vi "Delta Analysis.vi"() -> ()   [LabVIEW 2013]
uses:
  Common/Delta Analyzor/Workspace Scope.ctl
  <vilib>/Math Plots/3D Math Plots/3D Scatter/3D Scatter XCtrl/3D Scatter.xctl
  Common/Delta Analyzor/Delta Analyzor.lvclass
  <vilib>/Analysis/_algsub.llb/Real Vector Norm.vi
  <vilib>/picture/3D Picture Control/Object/Create Object (name).vi
  <vilib>/Math Plots/3D Math Plots/3D Scatter/3D Scatter Datatype/Public/Plot Helper (Vector).vi
  Common/Delta Robot Kinematics/Delta Robot Kinematics.lvclass
  <vilib>/Math Plots/3D Math Plots/3D Scatter/3D Scatter Datatype/3D Scatter Datatype.lvclass
  <vilib>/Analysis/NI_AALPro.lvlib
  <vilib>/picture/3D Picture Control/NI_3D Picture Control.lvlib
panel:
  out "number test points":i32
  out "XY Graph":cluster{dbl[], dbl[]}(graph)
  out "3D Scatter 2":refnum<class "3D Plot Datatype.lvclass">[](xcontrol)
  out "x*y":dbl[][](array[numeric])
  in  "stop":bool
  out "3D Picture":refnum<vi>(3d-picture)
  out "Waveform Chart":dbl[](graph)
  out "velocity time":u32
  out "workspace time (ms)":u32
  out "3D Scatter":refnum<class "3D Plot Datatype.lvclass">[](xcontrol)
  in  "Workspace Scope":T1={"X range"={"min"=-1.0, "max"=1.0}, "Y range"={"min"=-1.0, "max"=1.0}, "Z range"={"min"=-1.2, "max"=-0.2}}
  in  "XYZ Resolution":dbl[](array[numeric])=[0.05, 0.05, 0.05]
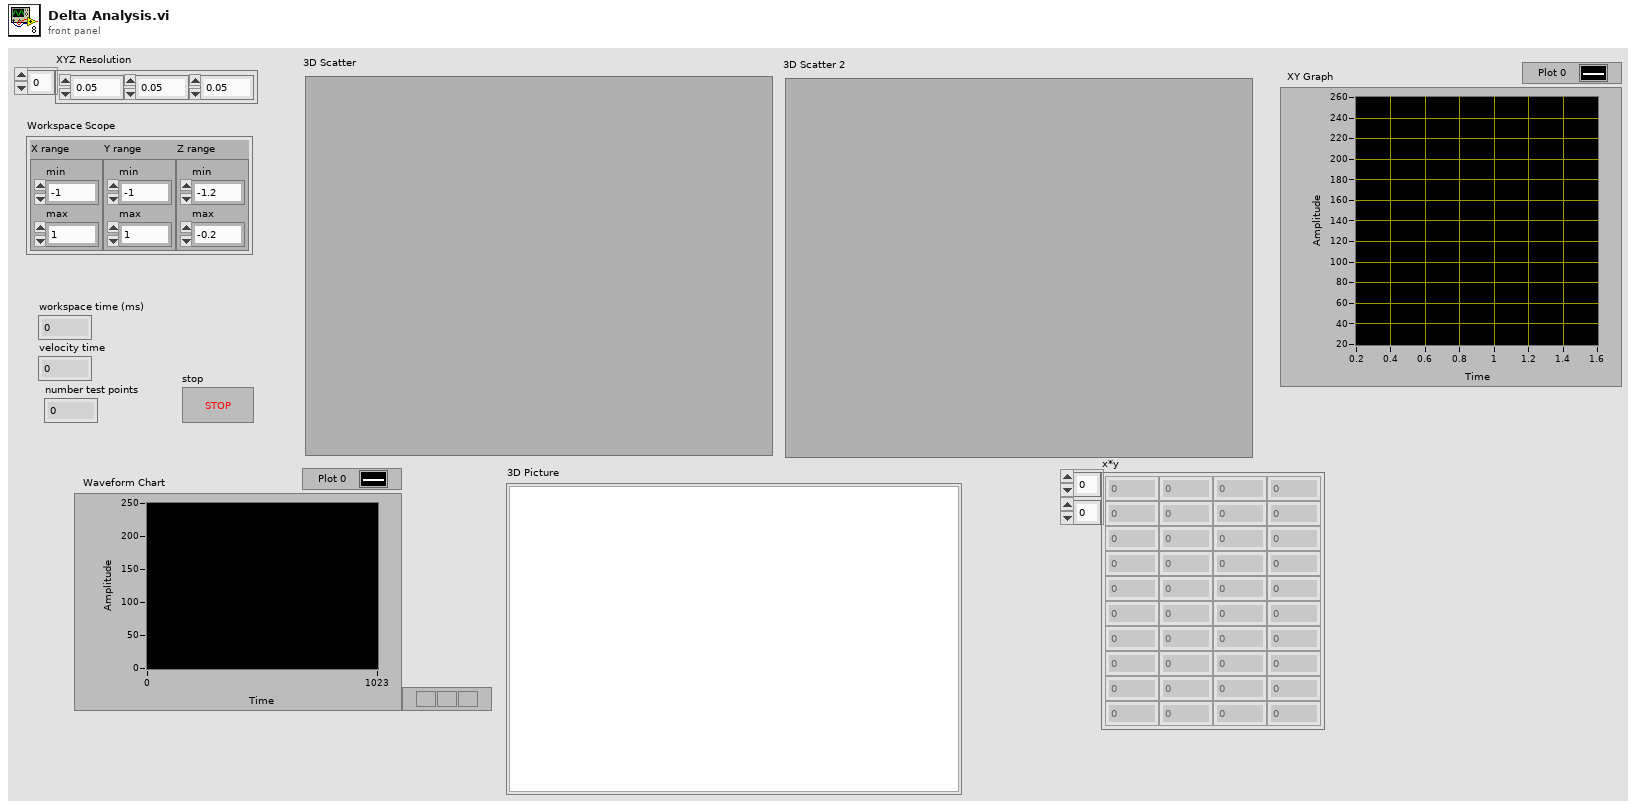
[diagram p1: front panel]
types:
  T1 = typedef "Delta Analyzor.lvclass/Workspace Scope.ctl" = cluster{"X range":cluster{"min":dbl, "max":dbl}, "Y range":cluster{"min":dbl, "max":dbl}, "Z range":cluster{"min":dbl, "max":dbl}}
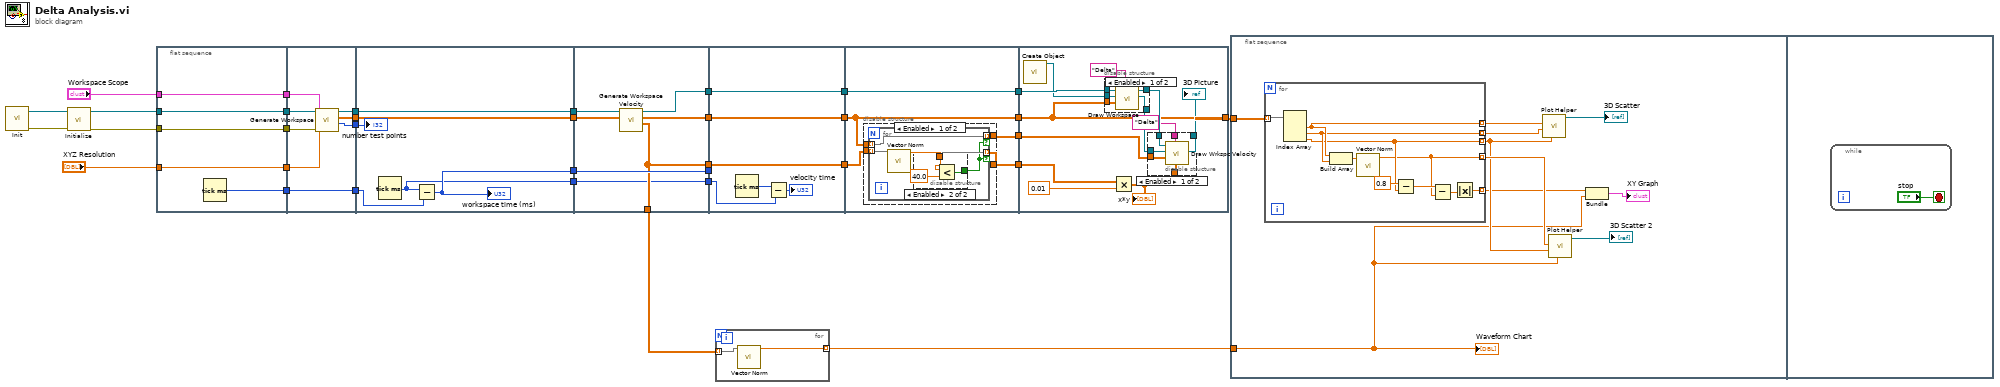
[diagram p0: block diagram]
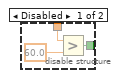
[diagram p2: hidden frame]
diagram:
  n1 = call "Init.vi"() -> ("error out"=w33:errorcluster, "Delta Robot Kin"=w34:refnum<class "Delta Robot Kinematics.lvclass">)  [unwired: 10 in]
  n2 = call "Initialize.vi"("error in (no error)"=w33, "Delta Robot Kinematics"=w34) -> ("error out"=w31:errorcluster, "Delta Analyzor out"=w32:refnum<class "Delta Analyzor.lvclass">)  [unwired: 8 in]
  n3 = flat-sequence {
    tunnel: "Workspace Scope" -> [w36]
    tunnel: "XYZ Resolution" -> [w37]
    tunnel: w31 -> [w38]
    tunnel: w32 -> [w39]
    tunnel: [w39] -> w28
    tunnel: [w38] -> w27
    tunnel: [w37] -> w26
    tunnel: [w36] -> w25
    tunnel: [w35] -> w23
    tunnel: w28 -> [w47]
    tunnel: w27 -> [w46]
    tunnel: w26 -> [w45]
    tunnel: w25 -> [w44]
    tunnel: [w43] -> w24
    tunnel: w23 -> [w42]
    tunnel: [w42] -> w22
    tunnel: [w41] -> w19
    tunnel: [w40] -> w8
    tunnel: w24 -> [w53]
    tunnel: w22 -> [w52]
    tunnel: [w53] -> w21
    tunnel: w19 -> [w51]
    tunnel: [w51] -> w18
    tunnel: [w50] -> w17
    tunnel: [w49] -> w9
    tunnel: w8 -> [w48]
    tunnel: w21 -> [w59]
    tunnel: [w58] -> w20
    tunnel: w18 -> [w60]
    tunnel: w17 -> [w57]
    tunnel: [w57] -> w16
    tunnel: [w55] -> w15
    tunnel: [w56] -> w12
    tunnel: [w55] -> w11
    tunnel: [w54] -> w10
    tunnel: w9 -> [w54]
    tunnel: w20 -> [w66]
    tunnel: w16 -> [_]
    tunnel: [w66] -> w7
    tunnel: w12 -> [w63]
    tunnel: [w63] -> w5
    tunnel: w11 -> [w62]
    tunnel: [w62] -> w3
    tunnel: w10 -> [w61]
    tunnel: w7 -> [w69]
    tunnel: [w69] -> w6
    tunnel: w5 -> [w71]
    tunnel: [w71] -> w4
    tunnel: w3 -> [w70]
    tunnel: [w67] -> w2
    tunnel: [w68] -> w1
    tunnel: [w94] -> w13
    tunnel: w6 -> [w94]
    tunnel: w4 -> [w99]
    tunnel: w2 -> [w91]
    tunnel: w1 -> [w88]
    frame #0 {
      n4 = Tick Count (ms)() -> (millisecond timer value=w35:u32)
    }
    frame #1 {
      n5 = call-dynamic "Generate Workspace.vi"("error in (no error)"=w46, "XYZ Resolution"=w45, "Workspace Scope"=w44, "Delta Analyzor in"=w47) -> ("number test points"=w40:i32, "workspace"=w43:dbl[][], "Delta Analyzor out"=w41:refnum<class "Delta Analyzor.lvclass">)  [unwired: 4 in, 1 out]
    }
    frame #2 {
      n6 = Tick Count (ms)() -> (millisecond timer value=w49:u32)
      n7 = Subtract(x=w49, y=w52) -> (x-y=w50:u32)
      "workspace time (ms)" <- w50
      "number test points" <- w48
    }
    frame #3 {
      n8 = call-dynamic "Generate Workspace Velocity.vi"("workspace in"=w59, "Delta Analyzor in"=w60) -> ("velocities"=w55:dbl[][], "workspace out"=w58:dbl[][], "Delta Analyzor out"=w56:refnum<class "Delta Analyzor.lvclass">)  [unwired: 6 in, 1 out]
    }
    frame #4 {
      n9 = Tick Count (ms)() -> (millisecond timer value=w65:u32)
      n10 = Subtract(x=w65, y=w61) -> (x-y=→"velocity time":u32)
    }
    frame #5 {
      n11 = disable-structure shown="Enabled" {
        disable-tunnel: w70 -> [w75 w86]
        disable-tunnel: w69 -> [w74 w87]
        disable-tunnel: [w73 w87] -> w68
        disable-tunnel: [w72 w86] -> w67
        frame Enabled {
          n12 = for {
            tunnel: w75 -> [w78] mode=indexing
            tunnel: w74 -> [w77] mode=indexing
            tunnel: [w78] -> w72 mode=indexing if=w76
            tunnel: [w77] -> w73 mode=indexing if=w76
            n13 = call-poly <vilib>:"Vector Norm.vi"("Input Vector"=w78) -> ("norm"=w79:dbl)  [unwired: 9 in, 1 out]
            n14 = disable-structure shown="Enabled" {
              disable-tunnel: w79 -> [w81 w85]
              disable-tunnel: [w80 w84] -> w76
              frame Disabled {
                n15 = Greater?(x=w81, y=60.0) -> (0:w80:bool)
              }
              frame Enabled {
                n16 = Less?(x=w85, y=40.0) -> (x < y?=w84:bool)
              }
            }
          }
        }
        frame Disabled {
        }
      }
    }
    frame #6 {
      n17 = call-poly <vilib>:"Create Object.vi"() -> ("Scene:New Object"=w98:refnum<vi>)  [unwired: 10 in, 1 out]
      n18 = disable-structure shown="Enabled" {
        disable-tunnel: w99 -> [w112 w113]
        disable-tunnel: w98 -> [w111 w114]
        disable-tunnel: "Delta" ("name") -> [w110 _]
        disable-tunnel: [w109 w113] -> w96
        disable-tunnel: [w108 w114] -> w95
        disable-tunnel: w94 -> [w107 _]
        frame Enabled {
          n19 = call-dynamic "Draw Workspace.vi"("name"=w110, "workspace in"=w107, "parent sence"=w111, "Delta Analyzor in"=w112) -> ("parent sence out"=w108:refnum<vi>, "Delta Analyzor out"=w109:refnum<class "Delta Analyzor.lvclass">)  [unwired: 4 in, 2 out]
        }
        frame Disabled {
        }
      }
      n20 = Multiply(x=w91, y=0.01) -> (x*y=w90:dbl[][])
      "x*y" <- w90
      n21 = disable-structure shown="Enabled" {
        disable-tunnel: w96 -> [w105 _]
        disable-tunnel: w95 -> [w104 w106]
        disable-tunnel: "Delta" ("name") -> [w103 _]
        disable-tunnel: [w102 w106] -> w92
        disable-tunnel: w90 -> [w101 _]
        disable-tunnel: w88 -> [w100 _]
        frame Enabled {
          n22 = call-dynamic "Draw Wrkspc Velocity.vi"("velocities"=w101, "name"=w103, "workspace in"=w100, "parent sence"=w104, "Delta Analyzor in"=w105) -> ("parent sence out"=w102:refnum<vi>)  [unwired: 3 in, 3 out]
        }
        frame Disabled {
        }
      }
      "3D Picture" <- w92
    }
  }
  n23 = for {
    tunnel: w15 -> [w116] mode=indexing
    tunnel: [w115] -> w14 mode=indexing
    n24 = call-poly <vilib>:"Vector Norm.vi"("Input Vector"=w116) -> ("norm"=w115:dbl)  [unwired: 9 in, 1 out]
  }
  n25 = flat-sequence {
    tunnel: w14 -> [w118]
    tunnel: w13 -> [w123]
    frame #0 {
      n26 = for {
        tunnel: w123 -> [w133] mode=indexing
        tunnel: [w136] -> w125 mode=indexing
        tunnel: [w135] -> w124 mode=indexing
        tunnel: [w129] -> w120 mode=indexing
        tunnel: [w128] -> w121 mode=indexing
        tunnel: [w132] -> w119 mode=indexing
        n27 = Index Array(array=w133) -> (element #1=w136:dbl, element #2=w135:dbl, element #3=w129:dbl)  [unwired: 3 in]
        n28 = Build Array(w136, w135) -> (w134:dbl[])
        n29 = call-poly <vilib>:"Vector Norm.vi"("Input Vector"=w134) -> ("norm"=w128:dbl)  [unwired: 9 in, 1 out]
        n30 = Subtract(x=0.8, y=w129) -> (x-y=w130:dbl)
        n31 = Subtract(x=w130, y=w128) -> (x-y=w127:dbl)
        n32 = Absolute Value(x=w127) -> (abs(x)=w132:dbl)
      }
      n33 = call-poly <vilib>:"Plot Helper.vi"("z vector"=w120, "y vector"=w124, "x vector"=w125) -> ("3D Plot lvclass Array out"=→"3D Scatter":refnum<class "3D Plot Datatype.lvclass">[])  [unwired: 3 in, 5 out]
      n34 = call-poly <vilib>:"Plot Helper.vi"("z vector"=w118, "y vector"=w120, "x vector"=w121) -> ("3D Plot lvclass Array out"=→"3D Scatter 2":refnum<class "3D Plot Datatype.lvclass">[])  [unwired: 3 in, 5 out]
      n35 = Bundle(w119, w118) -> (→"XY Graph":cluster{dbl[], dbl[]})  [unwired: 1 in]
      "Waveform Chart" <- w118
    }
    frame #1 {
      n36 = while {
        stop <- "stop" stop-if-true
      }
    }
  }
